vi "GetNetworkTime.vi"(8 "error in (no error)":errorcluster, 11 "NetworkPluginNone":refnum<class "NetworkPluginNone.lvclass">) -> (0 "error out":errorcluster, 3 "NetworkPluginNone":refnum<class "NetworkPluginNone.lvclass">)   [LabVIEW 2014, in "NetworkImpairmentPlugins.lvlib" / "NetworkPluginNone.lvclass"]
uses:
  NetworkPluginNone.lvclass
  NetworkImpairmentPluginBase_class/Accessors/Read TimeArray.vi
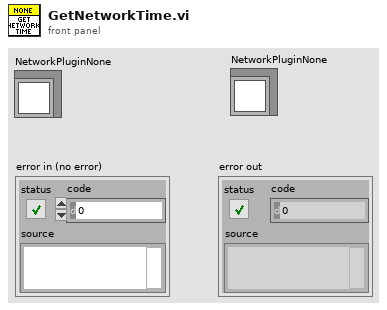
[diagram p1: front panel]
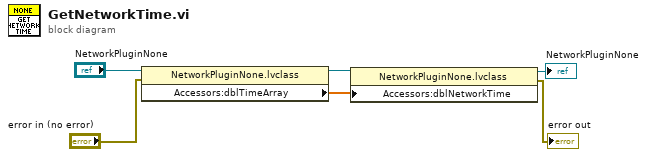
[diagram p0: block diagram]
diagram:
  n1 = property class="NetworkPluginNone.lvclass"(reference="NetworkPluginNone", error in="error in (no error)") -> (reference out=w4:refnum<class "NetworkPluginNone.lvclass">, "Accessors:dblTimeArray"=w3:dbl[])  [unwired: 1 out]
  n2 = property class="NetworkPluginNone.lvclass"(reference=w4, "Accessors:dblNetworkTime"=w3) -> (reference out=→"NetworkPluginNone":refnum<class "NetworkPluginNone.lvclass">, error out=→"error out":errorcluster)  [unwired: 1 in]
